vi "_RT Read XML Mass Range.vi"(4 "error in":errorcluster, 6 "# of MRs":i32, 7 "XML String":string) -> (0 "error out":errorcluster, 1 "Mass Range":T1[](array[typedef]) {"Res" items=["High/High", "Medium/Medium", "Low/Low", "High/Medium", "High/Low", "Medium/High", "Medium/Low", "Low/High", "Low/Medium"]}, 3 "Remaining String":string)   [LabVIEW 2015]
uses:
  Type/_Mass Range Property.ctl
  Type/_Mass Range Parameters.ctl
  Type/_RT Res Type.ctl
  Type/_XML Type.ctl
  _RT Global.vi
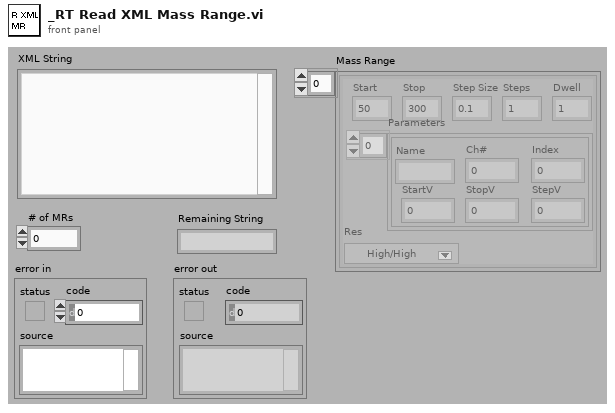
[diagram p1: front panel]
types:
  T1 = typedef "_Mass Range Property.ctl" = cluster{"Start":dbl, "Stop":dbl, "Step Size":dbl, "Steps":i32, "Dwell":dbl, "Parameters":T2[], "Res":T3}
  T2 = typedef "_Mass Range Parameters.ctl" = cluster{"Name":string, "Ch#":u8, "StartV":dbl, "StopV":dbl, "StepV":dbl, "Index":u8}
  T3 = typedef "_RT Res Type.ctl" = u16
  T4 = typedef "_XML Type.ctl" = enum16{"Configuration", "ConTable", "Method", "Experiment", "Mass Range", "Table", "LensTable", "ParamTable", "TuneParam", "MetParam", "MassRange", "LCMethod", "LCMethodFile", "RackType", "Vial", "PlatePos", "InjVol"}
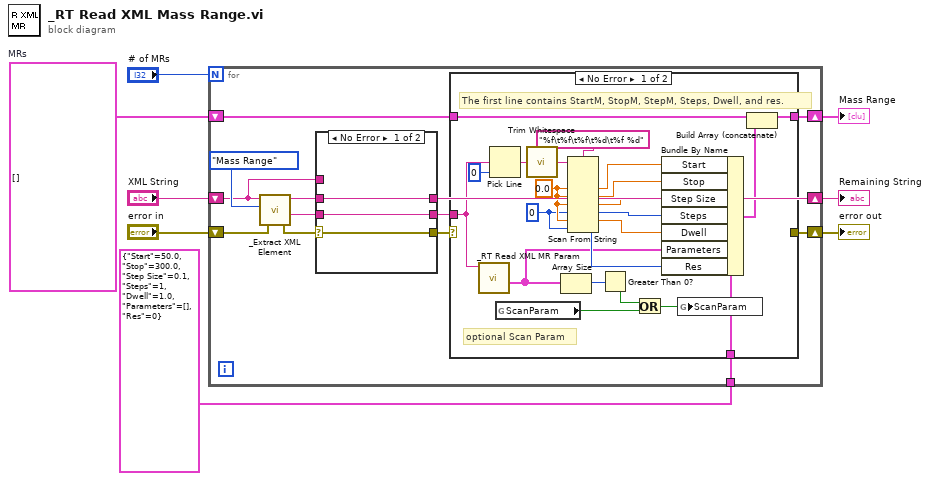
[diagram p0: block diagram]
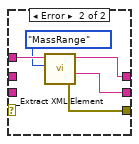
[diagram p2: hidden frame]
diagram:
  w3 = T1[] []  # MRs
  n1 = for {
    N: "# of MRs" -> [_]
    shift-right: [w10] -> w5
    shift-left: "XML String" -> [w9]
    shift-right: [w19] -> w4
    shift-left: "error in" -> [w20]
    shift-right: [w16] -> w1
    shift-left: w3 -> [w18]
    tunnel: T1 {"Start"=50.0, "Stop"=300.0, "Step Size"=0.1, "Steps"=1, "Dwell"=1.0, "Parameters"=[], "Res"=0} ("Mass Range") -> [w17]
    n2 = call "_Extract XML Element.vi"("error in"=w20, "XML Type"=_XML_Type."Mass Range", "XML String"=w9) -> ("error out"=w14:errorcluster, "Element"=w13:string, "Remaining String"=w11:string)  [unwired: 2 out]
    n3 = case shown="No Error" w14 {
      selector: w14 -> [w24 _]
      tunnel: [w24 w27] -> w15
      tunnel: w13 -> [w23 _]
      tunnel: [w23 w25] -> w12
      tunnel: w11 -> [w22 _]
      tunnel: [w22 w26] -> w10
      tunnel: w9 -> [_ w29]
      frame No Error {
      }
      frame Error {
        n4 = call "_Extract XML Element.vi"("XML Type"=_XML_Type."MassRange", "XML String"=w29) -> ("error out"=w27:errorcluster, "Element"=w25:string, "Remaining String"=w26:string)  [unwired: 1 in, 2 out]
      }
    }
    n5 = case shown="No Error" w15 {
      selector: w15 -> [_ w53]
      tunnel: [_ w53] -> w19
      tunnel: w12 -> [w46 _]
      tunnel: w18 -> [w40 w52]
      tunnel: w17 -> [w45 _]
      tunnel: [w38 w52] -> w16
      frame No Error {
        w47 = 0.0 ("Ch#")
        w36 = 0 ("Ch#")
        # "optional Scan Param"
        # "The first line contains StartM, StopM, StepM, Steps, Dwell, and res."
        n6 = call "_RT Read XML MR Param.vi"("XML String"=w46) -> ("Parameters"=w34:T2[])  [unwired: 4 in, 2 out]
        n7 = Pick Line(multi-line string=w46, line index=0) -> (output string=w51:string)  [unwired: 1 out]
        n8 = global read "_RT Global.vi" "ScanParam"() -> (w32:bool)
        n9 = call <vilib>:"Trim Whitespace.vi"("string"=w51) -> ("trimmed string"=w48:string)  [unwired: 1 in]
        n10 = Array Size(array=w34) -> (size(s)=w33:i32)
        n11 = Scan From String(format string="%f\t%f\t%f\t%d\t%f %d", input string=w48, default 1=w47, default 2=w47, default 3=w47, default 4=w36, default 5=w47, default 6=w36) -> (output 1=w44:dbl, output 2=w43:dbl, output 3=w42:dbl, output 4=w41:i32, output 5=w37:dbl, output 6=w35:i32)  [unwired: 2 in, 3 out]
        n12 = Greater Than 0?(x=w33) -> (x > 0?=w31:bool)
        n13 = Or(x=w31, y=w32) -> (x .or. y?=w30:bool)
        n14 = Bundle By Name(cluster=w45, "Start"=w44, "Stop"=w43, "Step Size"=w42, "Steps"=w41, "Dwell"=w37, "Parameters"=w34, "Res"=w35) -> (w39:T1)
        n15 = global write "_RT Global.vi" "ScanParam"(w30) -> ()
        n16 = Build Array (concatenate)(w40, w39) -> (w38:T1[])
      }
      frame Error {
      }
    }
  }
  "Remaining String" <- w5
  "error out" <- w4
  "Mass Range" <- w1
